vi "GenerateFilenames.vi"(8 "file number":i32, 10 "filename":string, 11 "Path":path) -> (3 "Filepath":path)   [LabVIEW 2019]
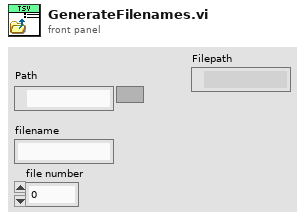
[diagram p1: front panel]
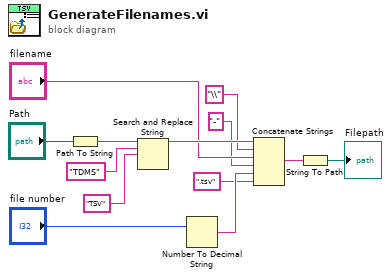
[diagram p0: block diagram]
diagram:
  n1 = Path To String(path="Path") -> (string=w13:string)
  n2 = Search and Replace String(input string=w13, search string="TDMS" ("input string"), replace string="TSV" ("replace string (\"\")")) -> (result string=w9:string)  [unwired: 5 in, 3 out]
  n3 = Number To Decimal String(number="file number") -> (decimal integer string=w5:string)  [unwired: 1 in]
  n4 = Concatenate Strings(w9, "\\" ("string"), "filename", "-" ("string"), w5, ".tsv" ("string")) -> (w2:string)
  n5 = String To Path(string=w2) -> (path=→"Filepath":path)
